vi "Collision Detection.vi"(2 "Map Entity Objects Positions":T3(array[cluster]), 3 "Max Player ID number":i32, 4 "Moving Object":T2) -> (0 "Bullet hit Player No.":i32, 1 "New Vector":T1)   [LabVIEW 2021]
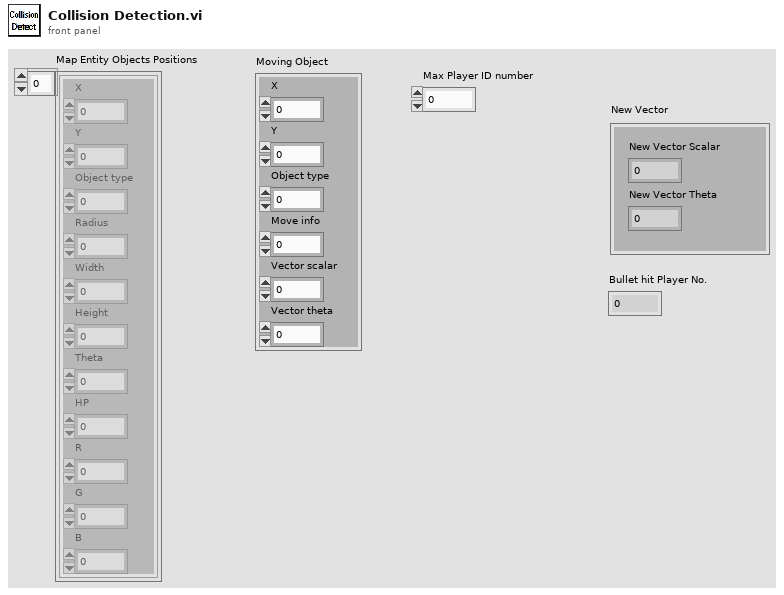
[diagram p1: front panel]
types:
  T1 = cluster{"New Vector Scalar":dbl, "New Vector Theta":dbl}
  T2 = cluster{"X":dbl, "Y":dbl, "Object type":dbl, "Move info":dbl, "Vector scalar":dbl, "Vector theta":dbl}
  T3 = cluster{"X":dbl, "Y":dbl, "Object type":dbl, "Radius":dbl, "Width":dbl, "Height":dbl, "Theta":dbl, "HP":dbl, "R":dbl, "G":dbl, "B":dbl}[]
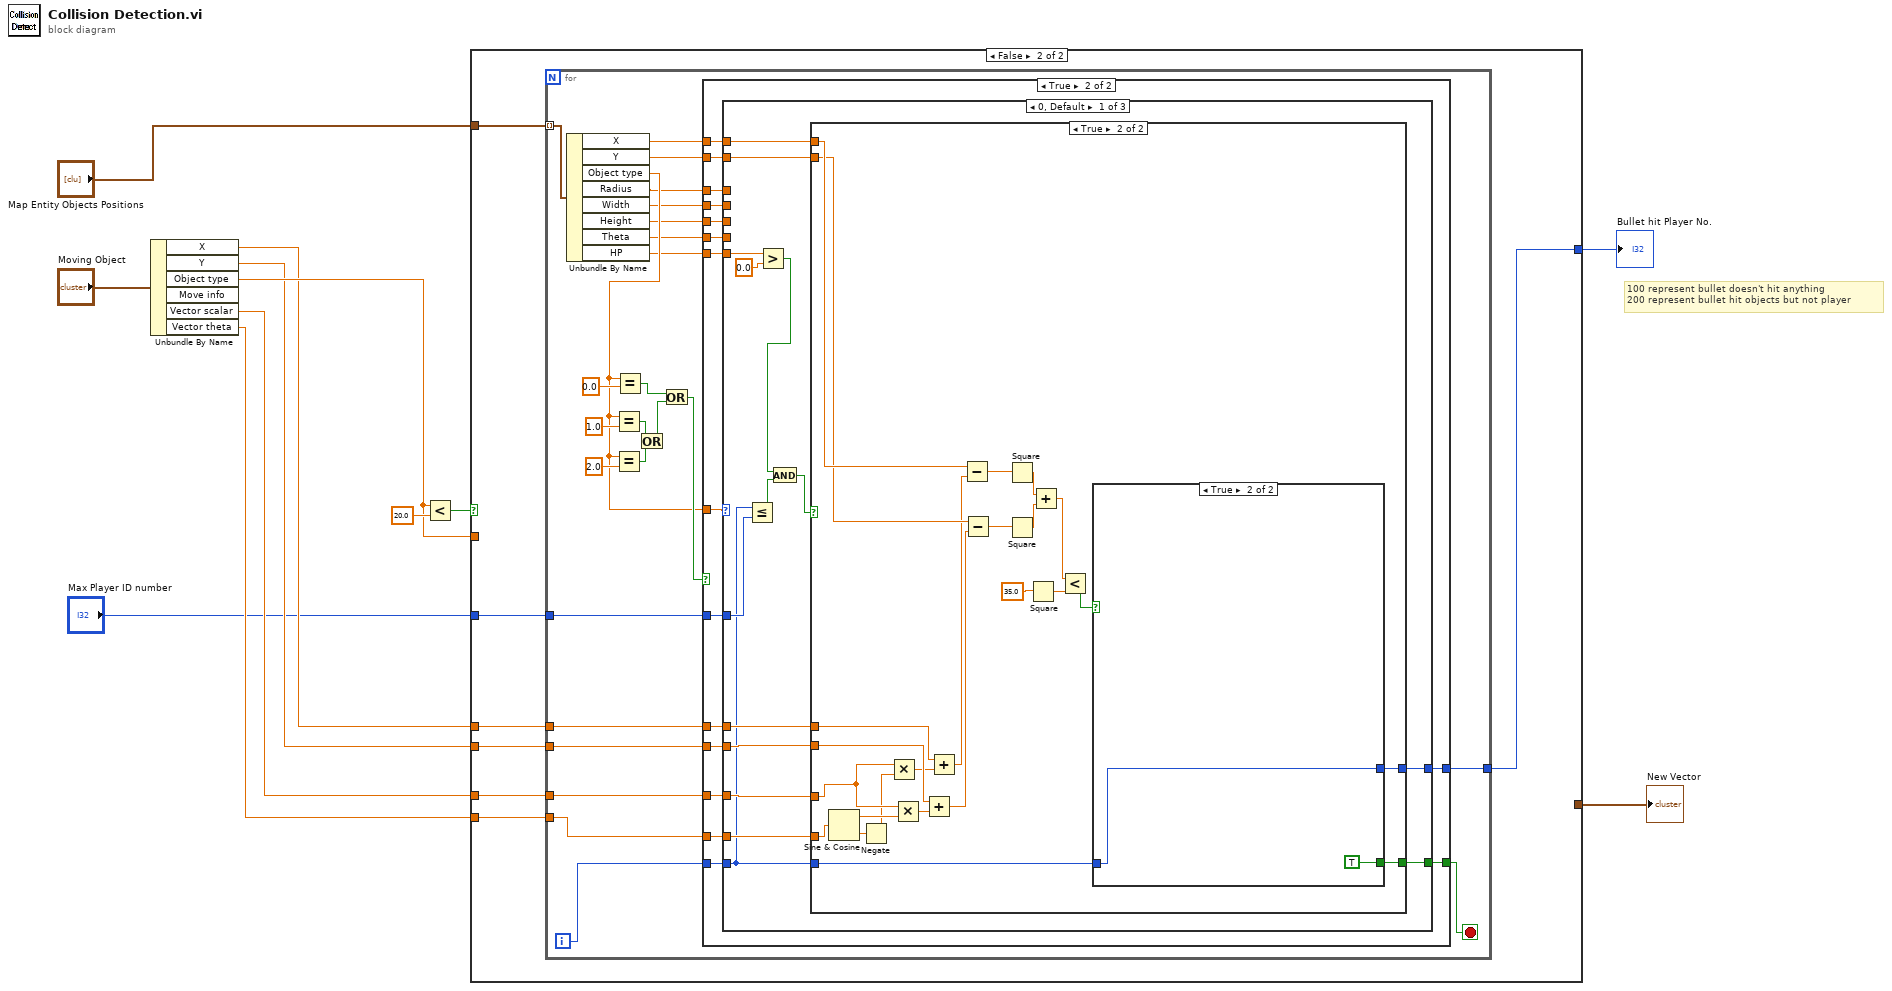
[diagram p0: block diagram]
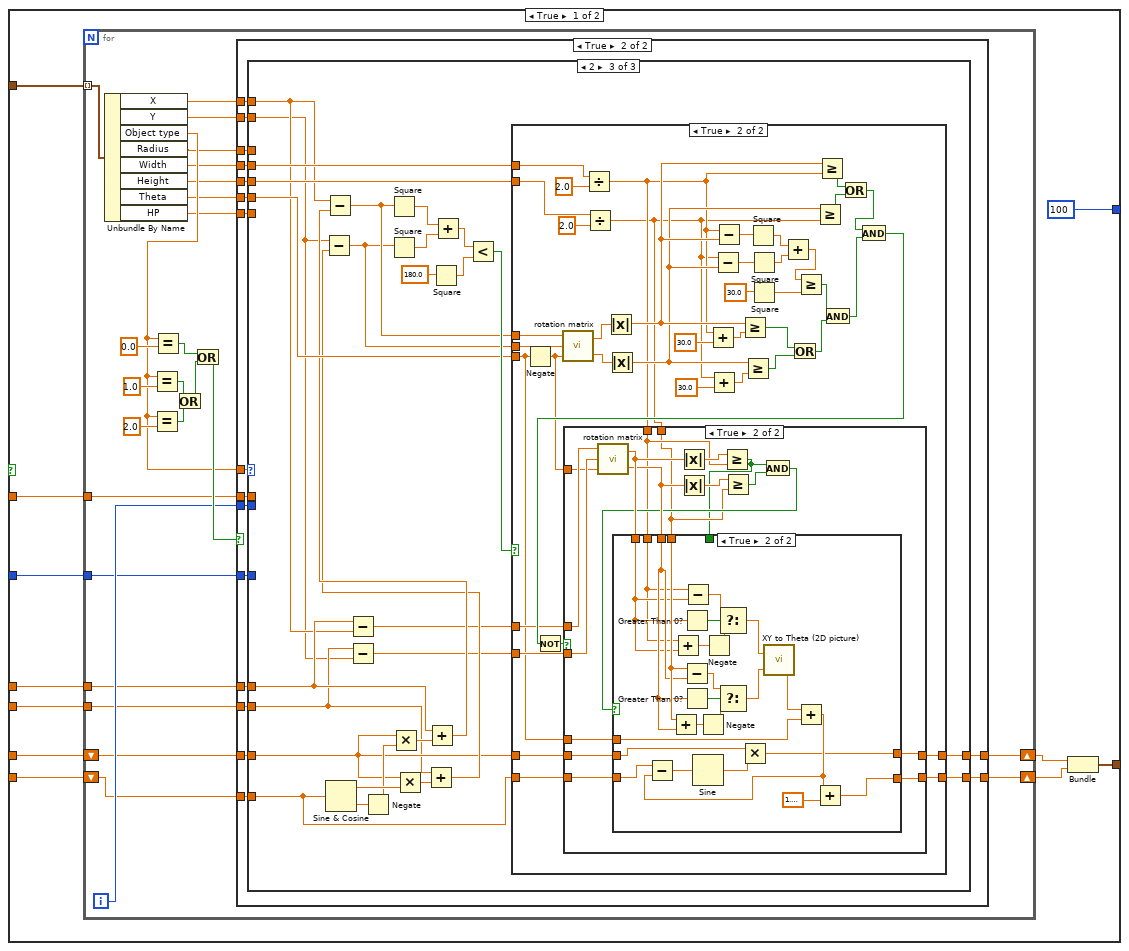
[diagram p2: hidden frame]
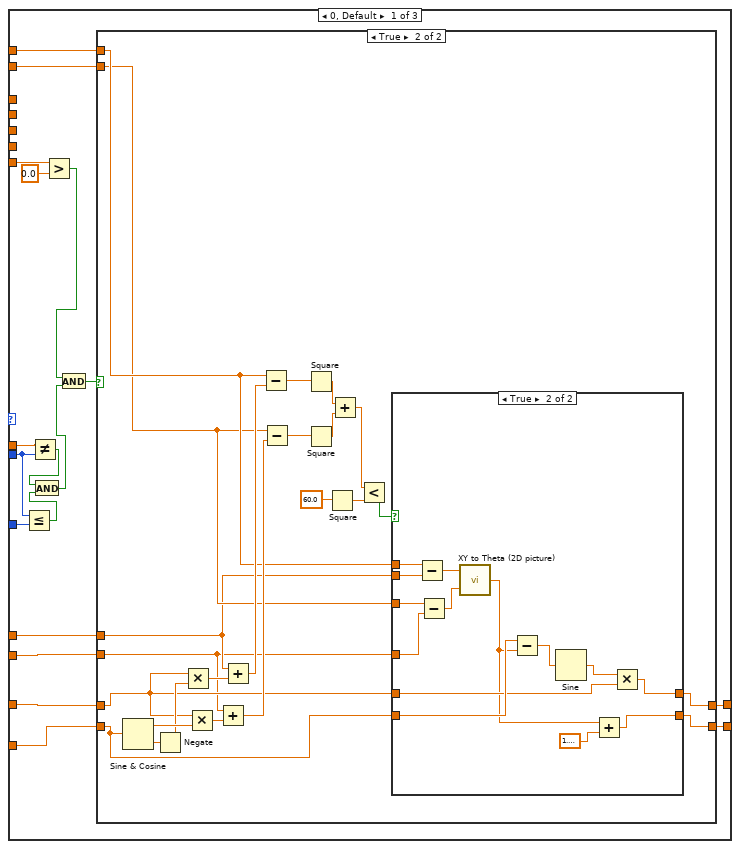
[diagram p4: hidden frame]
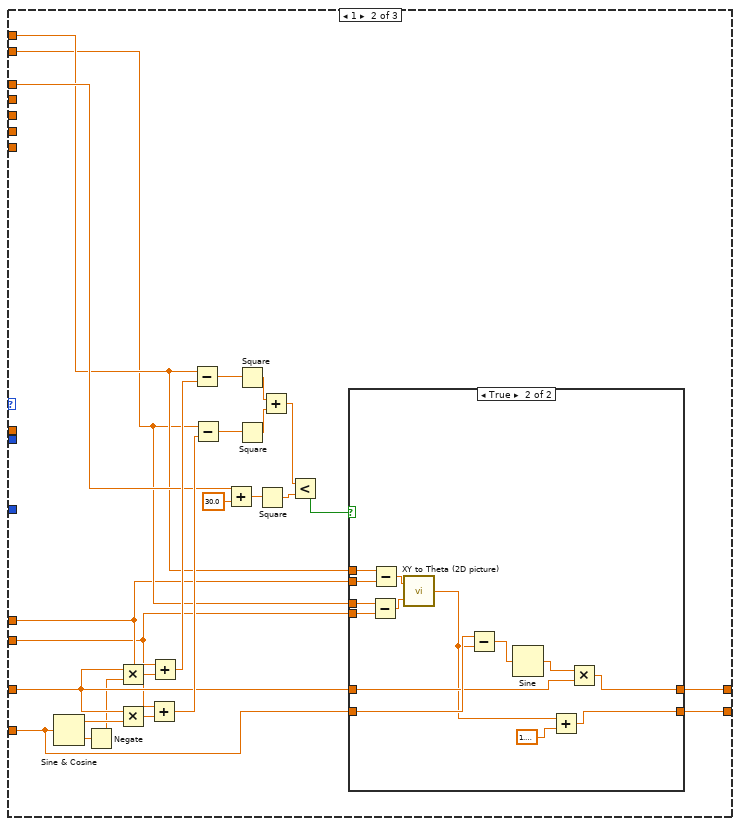
[diagram p7: hidden frame]
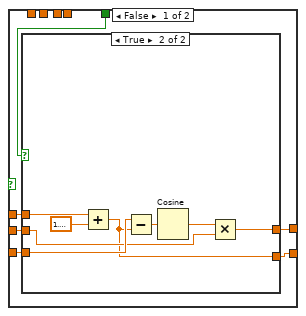
[diagram p11: hidden frame]
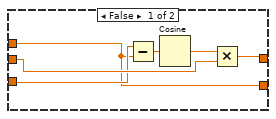
[diagram p12: hidden frame]
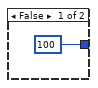
[diagram p13: hidden frame]
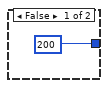
[diagram p14: hidden frame]
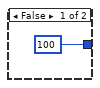
[diagram p15: hidden frame]
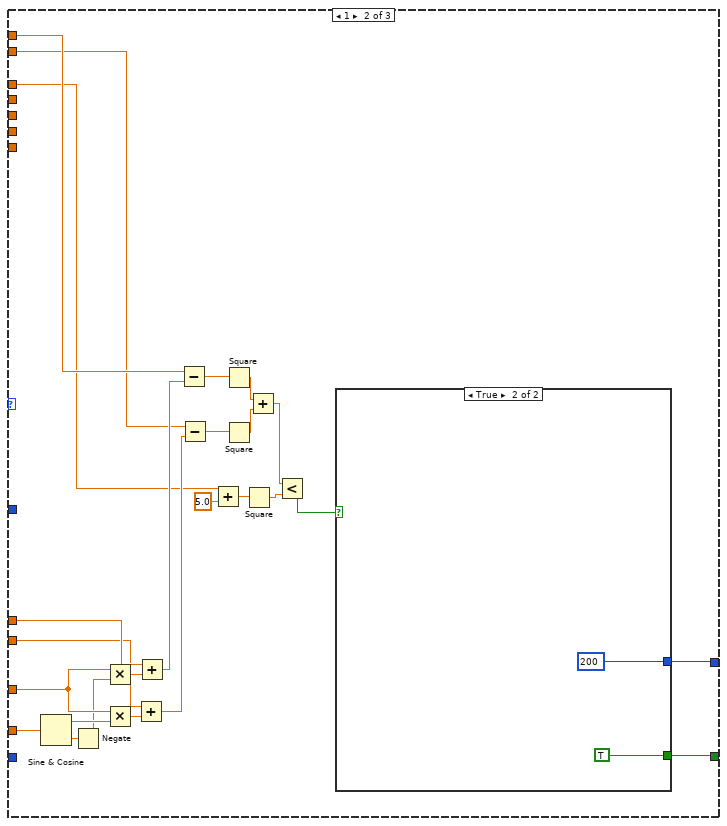
[diagram p16: hidden frame]
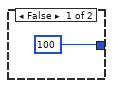
[diagram p17: hidden frame]
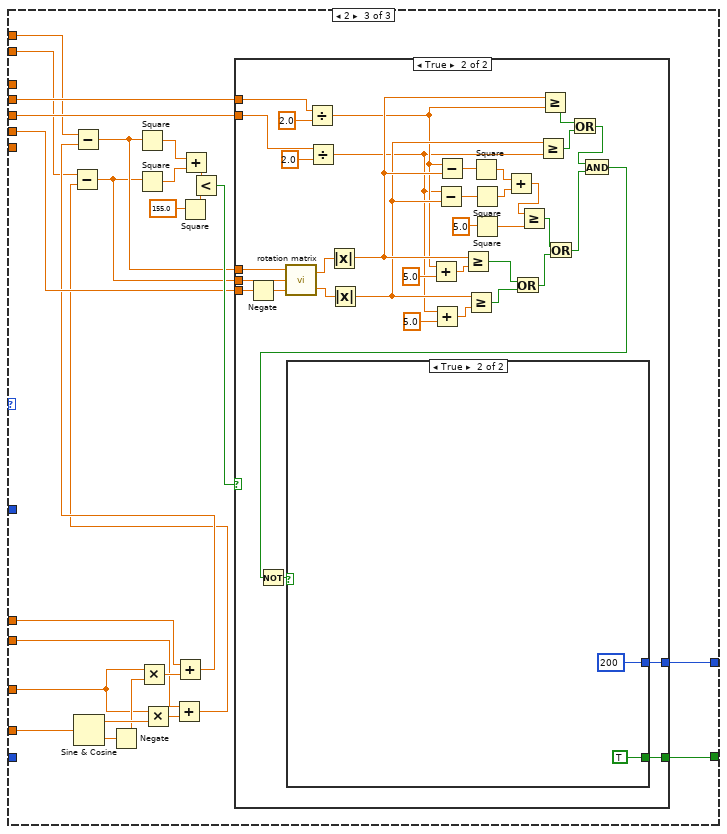
[diagram p18: hidden frame]
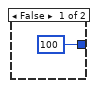
[diagram p19: hidden frame]
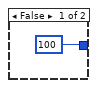
[diagram p20: hidden frame]
diagram:
  # "100 represent bullet doesn't hit anything\n200 represent bullet hit objects but not player"
  n1 = Unbundle By Name("Moving Object") -> ("X"=w4:dbl, "Y"=w3:dbl, "Object type"=w7:dbl, "Vector scalar"=w6:dbl, "Vector theta"=w5:dbl)  [unwired: 1 out]
  n2 = Less?(x=w7, y=20.0) -> (x < y?=w10:bool)
  n3 = case shown="False" w10 {
    tunnel: "Map Entity Objects Positions" -> [w23 w309]
    tunnel: [100 ("Bullet hit Player No.") w304] -> w8
    tunnel: w7 -> [w21 _]
    tunnel: w6 -> [w20 w308]
    tunnel: w5 -> [w19 w307]
    tunnel: w4 -> [w18 w306]
    tunnel: w3 -> [w17 w305]
    tunnel: [w14 _] -> w2
    tunnel: "Max Player ID number" -> [w13 w303]
    frame True {
      n4 = for {
        tunnel: w23 -> [w49] mode=indexing
        tunnel: w21 -> [w38]
        tunnel: w18 -> [w35]
        tunnel: w17 -> [w34]
        shift-right: [w30] -> w16
        shift-left: w20 -> [w36]
        shift-right: [w29] -> w15
        shift-left: w19 -> [w37]
        tunnel: w13 -> [w25]
        i -> [w39]
        n5 = Unbundle By Name(w49) -> ("X"=w33:dbl, "Y"=w32:dbl, "Object type"=w40:dbl, "Radius"=w31:dbl, "Width"=w28:dbl, "Height"=w27:dbl, "Theta"=w26:dbl, "HP"=w24:dbl)
        n6 = Equal?(x=w40, y=1.0) -> (x = y?=w45:bool)
        n7 = Equal?(x=w40, y=2.0) -> (x = y?=w44:bool)
        n8 = Equal?(x=w40, y=0.0) -> (x = y?=w43:bool)
        n9 = Or(x=w45, y=w44) -> (x .or. y?=w42:bool)
        n10 = Or(x=w43, y=w42) -> (x .or. y?=w41:bool)
        n11 = case shown="True" w41 {
          tunnel: w40 -> [_ w68]
          tunnel: w39 -> [_ w67]
          tunnel: w38 -> [_ w66]
          tunnel: w37 -> [w50 w65]
          tunnel: w36 -> [w51 w64]
          tunnel: w35 -> [_ w63]
          tunnel: w34 -> [_ w62]
          tunnel: w33 -> [_ w61]
          tunnel: w32 -> [_ w60]
          tunnel: w31 -> [_ w59]
          tunnel: [w51 w58] -> w30
          tunnel: [w50 w57] -> w29
          tunnel: w28 -> [_ w56]
          tunnel: w27 -> [_ w55]
          tunnel: w26 -> [_ w54]
          tunnel: w25 -> [_ w53]
          tunnel: w24 -> [_ w52]
          frame False {
          }
          frame True {
            n12 = case shown="2" w68 {
              tunnel: w67 -> [w75 _ _]
              tunnel: w66 -> [w86 _ _]
              tunnel: w65 -> [w82 w138 w176]
              tunnel: w64 -> [w84 w140 w175]
              tunnel: w63 -> [w80 w129 w172]
              tunnel: w62 -> [w81 w128 w170]
              tunnel: w61 -> [w79 w131 w171]
              tunnel: w60 -> [w78 w130 w169]
              tunnel: w59 -> [_ w143 _]
              tunnel: [w85 w141 w190] -> w58
              tunnel: [w83 w139 w189] -> w57
              tunnel: w56 -> [_ _ w178]
              tunnel: w55 -> [_ _ w177]
              tunnel: w54 -> [_ _ w186]
              tunnel: w53 -> [w74 _ _]
              tunnel: w52 -> [w73 _ _]
              frame 0, Default {
                n13 = Less Or Equal?(x=w75, y=w74) -> (x <= y?=w76:bool)
                n14 = Not Equal?(x=w86, y=w75) -> (x != y?=w77:bool)
                n15 = And(x=w77, y=w76) -> (x .and. y?=w69:bool)
                n16 = Greater?(x=w73, y=0.0) -> (0:w70:bool)
                n17 = And(x=w70, y=w69) -> (x .and. y?=w71:bool)
                n18 = case shown="True" w71 {
                  tunnel: [w88 w96] -> w85
                  tunnel: w84 -> [w88 w97]
                  tunnel: [w87 w95] -> w83
                  tunnel: w82 -> [w87 w98]
                  tunnel: w81 -> [_ w89]
                  tunnel: w80 -> [_ w90]
                  tunnel: w79 -> [_ w92]
                  tunnel: w78 -> [_ w91]
                  frame False {
                  }
                  frame True {
                    n19 = Sine & Cosine(0:w98) -> (1:w111:dbl, 2:w100:dbl)
                    n20 = Negate(x=w100) -> (-x=w99:dbl)
                    n21 = Multiply(x=w97, y=w99) -> (x*y=w109:dbl)
                    n22 = Multiply(x=w97, y=w111) -> (x*y=w110:dbl)
                    n23 = Add(x=w89, y=w110) -> (x+y=w108:dbl)
                    n24 = Add(x=w90, y=w109) -> (x+y=w107:dbl)
                    n25 = Subtract(x=w92, y=w107) -> (x-y=w102:dbl)
                    n26 = Subtract(x=w91, y=w108) -> (x-y=w101:dbl)
                    n27 = Square(x=w102) -> (x^2=w105:dbl)
                    n28 = Square(x=w101) -> (x^2=w106:dbl)
                    n29 = Square(x=60.0 ("y")) -> (x^2=w94:dbl)
                    n30 = Add(x=w105, y=w106) -> (x+y=w104:dbl)
                    n31 = Less?(x=w104, y=w94) -> (x < y?=w103:bool)
                    n32 = case shown="True" w103 {
                      tunnel: [w113 w126] -> w96
                      tunnel: w97 -> [w113 w123]
                      tunnel: [w112 w120] -> w95
                      tunnel: w98 -> [w112 w127]
                      tunnel: w92 -> [_ w117]
                      tunnel: w91 -> [_ w116]
                      tunnel: w90 -> [_ w115]
                      tunnel: w89 -> [_ w114]
                      frame False {
                      }
                      frame True {
                        n33 = Subtract(x=w117, y=w115) -> (x-y=w119:dbl)
                        n34 = Subtract(x=w116, y=w114) -> (x-y=w118:dbl)
                        n35 = call "XY to Theta (2D picture).vi"("y"=w118, "x"=w119) -> ("Theta"=w121:dbl)
                        n36 = Subtract(x=w127, y=w121) -> (x-y=w124:dbl)
                        n37 = Sine(x=w124) -> (sin(x)=w125:dbl)
                        n38 = Add(x=w121, y=1.5707963267948966) -> (x+y=w120:dbl)
                        n39 = Multiply(x=w125, y=w123) -> (x*y=w126:dbl)
                      }
                    }
                  }
                }
              }
              frame 1 {
                n40 = Sine & Cosine(0:w138) -> (1:w152:dbl, 2:w135:dbl)
                n41 = Negate(x=w135) -> (-x=w134:dbl)
                n42 = Multiply(x=w140, y=w134) -> (x*y=w150:dbl)
                n43 = Multiply(x=w140, y=w152) -> (x*y=w151:dbl)
                n44 = Add(x=w128, y=w151) -> (x+y=w149:dbl)
                n45 = Add(x=w129, y=w150) -> (x+y=w148:dbl)
                n46 = Subtract(x=w131, y=w148) -> (x-y=w137:dbl)
                n47 = Subtract(x=w130, y=w149) -> (x-y=w136:dbl)
                n48 = Add(x=w143, y=30.0) -> (x+y=w132:dbl)
                n49 = Square(x=w137) -> (x^2=w146:dbl)
                n50 = Square(x=w136) -> (x^2=w147:dbl)
                n51 = Square(x=w132) -> (x^2=w133:dbl)
                n52 = Add(x=w146, y=w147) -> (x+y=w145:dbl)
                n53 = Less?(x=w145, y=w133) -> (x < y?=w142:bool)
                n54 = case shown="True" w142 {
                  tunnel: [w154 w167] -> w141
                  tunnel: w140 -> [w154 w164]
                  tunnel: [w153 w161] -> w139
                  tunnel: w138 -> [w153 w168]
                  tunnel: w131 -> [_ w158]
                  tunnel: w130 -> [_ w157]
                  tunnel: w129 -> [_ w156]
                  tunnel: w128 -> [_ w155]
                  frame False {
                  }
                  frame True {
                    n55 = Subtract(x=w157, y=w155) -> (x-y=w160:dbl)
                    n56 = Subtract(x=w158, y=w156) -> (x-y=w159:dbl)
                    n57 = call "XY to Theta (2D picture).vi"("y"=w160, "x"=w159) -> ("Theta"=w162:dbl)
                    n58 = Subtract(x=w168, y=w162) -> (x-y=w165:dbl)
                    n59 = Sine(x=w165) -> (sin(x)=w166:dbl)
                    n60 = Add(x=w162, y=1.5707963267948966) -> (x+y=w161:dbl)
                    n61 = Multiply(x=w166, y=w164) -> (x*y=w167:dbl)
                  }
                }
              }
              frame 2 {
                n62 = Sine & Cosine(0:w176) -> (1:w185:dbl, 2:w182:dbl)
                n63 = Subtract(x=w172, y=w171) -> (x-y=w174:dbl)
                n64 = Subtract(x=w170, y=w169) -> (x-y=w173:dbl)
                n65 = Negate(x=w182) -> (-x=w181:dbl)
                n66 = Multiply(x=w175, y=w181) -> (x*y=w183:dbl)
                n67 = Multiply(x=w175, y=w185) -> (x*y=w184:dbl)
                n68 = Add(x=w170, y=w184) -> (x+y=w179:dbl)
                n69 = Subtract(x=w169, y=w179) -> (x-y=w187:dbl)
                n70 = Square(x=w187) -> (x^2=w196:dbl)
                n71 = Add(x=w172, y=w183) -> (x+y=w180:dbl)
                n72 = Subtract(x=w171, y=w180) -> (x-y=w188:dbl)
                n73 = Square(x=w188) -> (x^2=w195:dbl)
                n74 = Square(x=180.0 ("y")) -> (x^2=w192:dbl)
                n75 = Add(x=w195, y=w196) -> (x+y=w194:dbl)
                n76 = Less?(x=w194, y=w192) -> (x < y?=w191:bool)
                n77 = case shown="True" w191 {
                  tunnel: [w198 w212] -> w190
                  tunnel: w175 -> [w198 w211]
                  tunnel: [w197 w210] -> w189
                  tunnel: w176 -> [w197 w209]
                  tunnel: w188 -> [_ w239]
                  tunnel: w187 -> [_ w238]
                  tunnel: w186 -> [_ w203]
                  tunnel: w178 -> [_ w235]
                  tunnel: w177 -> [_ w234]
                  tunnel: w174 -> [_ w208]
                  tunnel: w173 -> [_ w207]
                  frame False {
                  }
                  frame True {
                    n78 = Negate(x=w203) -> (-x=w206:dbl)
                    n79 = call "rotation matrix.vi"("angle"=w206, "y"=w238, "x"=w239) -> ("new y"=w232:dbl, "new x"=w233:dbl)
                    n80 = Divide(x=w235, y=2.0) -> (x/y=w205:dbl)
                    n81 = Divide(x=w234, y=2.0) -> (x/y=w204:dbl)
                    n82 = Absolute Value(x=w233) -> (abs(x)=w216:dbl)
                    n83 = Absolute Value(x=w232) -> (abs(x)=w215:dbl)
                    n84 = Add(x=w205, y=30.0) -> (x+y=w226:dbl)
                    n85 = Add(x=w204, y=30.0) -> (x+y=w227:dbl)
                    n86 = Subtract(x=w204, y=w215) -> (x-y=w217:dbl)
                    n87 = Subtract(x=w205, y=w216) -> (x-y=w218:dbl)
                    n88 = Greater Or Equal?(x=w216, y=w226) -> (x >= y?=w231:bool)
                    n89 = Greater Or Equal?(x=w215, y=w227) -> (x >= y?=w230:bool)
                    n90 = Square(x=w218) -> (x^2=w221:dbl)
                    n91 = Square(x=w217) -> (x^2=w220:dbl)
                    n92 = Square(x=30.0 ("y")) -> (x^2=w225:dbl)
                    n93 = Add(x=w221, y=w220) -> (x+y=w219:dbl)
                    n94 = Or(x=w231, y=w230) -> (x .or. y?=w199:bool)
                    n95 = Greater Or Equal?(x=w219, y=w225) -> (x >= y?=w223:bool)
                    n96 = Greater Or Equal?(x=w215, y=w204) -> (x >= y?=w202:bool)
                    n97 = Greater Or Equal?(x=w216, y=w205) -> (x >= y?=w201:bool)
                    n98 = And(x=w223, y=w199) -> (x .and. y?=w222:bool)
                    n99 = Or(x=w201, y=w202) -> (x .or. y?=w200:bool)
                    n100 = And(x=w200, y=w222) -> (x .and. y?=w213:bool)
                    n101 = Not(x=w213) -> (.not. x?=w214:bool)
                    n102 = case shown="True" w214 {
                      tunnel: [w241 w245] -> w212
                      tunnel: w211 -> [w241 w243]
                      tunnel: [w240 w246] -> w210
                      tunnel: w209 -> [w240 w244]
                      tunnel: w208 -> [_ w258]
                      tunnel: w207 -> [_ w257]
                      tunnel: w206 -> [_ w256]
                      tunnel: w205 -> [_ w249]
                      tunnel: w204 -> [_ w248]
                      tunnel: w203 -> [_ w247]
                      frame False {
                      }
                      frame True {
                        n103 = call "rotation matrix.vi"("angle"=w256, "y"=w257, "x"=w258) -> ("new y"=w254:dbl, "new x"=w255:dbl)
                        n104 = Absolute Value(x=w255) -> (abs(x)=w250:dbl)
                        n105 = Absolute Value(x=w254) -> (abs(x)=w251:dbl)
                        n106 = Greater Or Equal?(x=w250, y=w249) -> (x >= y?=w242:bool)
                        n107 = Greater Or Equal?(x=w251, y=w248) -> (x >= y?=w253:bool)
                        n108 = And(x=w242, y=w253) -> (x .and. y?=w252:bool)
                        n109 = case shown="True" w252 {
                          tunnel: w254 -> [_ w297]
                          tunnel: w248 -> [_ w298]
                          tunnel: w255 -> [_ w296]
                          tunnel: w249 -> [_ w282]
                          tunnel: w247 -> [w263 w292]
                          tunnel: [w259 w290] -> w246
                          tunnel: [w260 w284] -> w245
                          tunnel: w244 -> [w262 w289]
                          tunnel: w243 -> [w261 w285]
                          tunnel: w242 -> [w264 _]
                          frame False {
                            n110 = case shown="True" w264 {
                              tunnel: w263 -> [w265 w277]
                              tunnel: w262 -> [w266 w276]
                              tunnel: w261 -> [w267 w274]
                              tunnel: [w268 w272] -> w260
                              tunnel: [w265 w271] -> w259
                              frame False {
                                n111 = Subtract(x=w266, y=w265) -> (x-y=w270:dbl)
                                n112 = Cosine(x=w270) -> (cos(x)=w269:dbl)
                                n113 = Multiply(x=w269, y=w267) -> (x*y=w268:dbl)
                              }
                              frame True {
                                n114 = Add(x=w277, y=1.5707963267948966) -> (x+y=w271:dbl)
                                n115 = Subtract(x=w276, y=w271) -> (x-y=w275:dbl)
                                n116 = Cosine(x=w275) -> (cos(x)=w273:dbl)
                                n117 = Multiply(x=w273, y=w274) -> (x*y=w272:dbl)
                              }
                            }
                          }
                          frame True {
                            n118 = Add(x=w298, y=w297) -> (x+y=w280:dbl)
                            n119 = Add(x=w282, y=w296) -> (x+y=w279:dbl)
                            n120 = Greater Than 0?(x=w296) -> (x > 0?=w299:bool)
                            n121 = Subtract(x=w298, y=w297) -> (x-y=w302:dbl)
                            n122 = Greater Than 0?(x=w297) -> (x > 0?=w300:bool)
                            n123 = Subtract(x=w282, y=w296) -> (x-y=w301:dbl)
                            n124 = Negate(x=w280) -> (-x=w281:dbl)
                            n125 = Negate(x=w279) -> (-x=w283:dbl)
                            n126 = Select(t=w301, s=w299, f=w283) -> (s? t:f=w295:dbl)
                            n127 = Select(t=w302, s=w300, f=w281) -> (s? t:f=w294:dbl)
                            n128 = call "XY to Theta (2D picture).vi"("y"=w294, "x"=w295) -> ("Theta"=w293:dbl)
                            n129 = Add(x=w293, y=w292) -> (x+y=w288:dbl)
                            n130 = Subtract(x=w289, y=w288) -> (x-y=w287:dbl)
                            n131 = Sine(x=w287) -> (sin(x)=w286:dbl)
                            n132 = Multiply(x=w285, y=w286) -> (x*y=w284:dbl)
                            n133 = Add(x=w288, y=1.5707963267948966) -> (x+y=w290:dbl)
                          }
                        }
                      }
                    }
                  }
                }
              }
            }
          }
        }
      }
      n134 = Bundle("Vector scalar"=w16, "Vector theta"=w15) -> (w14:cluster{"Vector scalar":dbl, "Vector theta":dbl})  [unwired: 1 in]
    }
    frame False {
      n135 = for {
        tunnel: w309 -> [w334] mode=indexing
        tunnel: w306 -> [w322]
        tunnel: w305 -> [w321]
        tunnel: w308 -> [w323]
        tunnel: w307 -> [w324]
        tunnel: [w312] -> w304
        tunnel: w303 -> [w311]
        i -> [w313]
        stop <- w314 stop-if-true
        n136 = Unbundle By Name(w334) -> ("X"=w320:dbl, "Y"=w319:dbl, "Object type"=w325:dbl, "Radius"=w318:dbl, "Width"=w317:dbl, "Height"=w316:dbl, "Theta"=w315:dbl, "HP"=w310:dbl)
        n137 = Equal?(x=w325, y=1.0) -> (x = y?=w330:bool)
        n138 = Equal?(x=w325, y=2.0) -> (x = y?=w329:bool)
        n139 = Equal?(x=w325, y=0.0) -> (x = y?=w328:bool)
        n140 = Or(x=w330, y=w329) -> (x .or. y?=w327:bool)
        n141 = Or(x=w328, y=w327) -> (x .or. y?=w326:bool)
        n142 = case shown="True" w326 {
          tunnel: w325 -> [_ w351]
          tunnel: w324 -> [_ w350]
          tunnel: w323 -> [_ w349]
          tunnel: w322 -> [_ w348]
          tunnel: w321 -> [_ w347]
          tunnel: w320 -> [_ w346]
          tunnel: w319 -> [_ w345]
          tunnel: w318 -> [_ w344]
          tunnel: w317 -> [_ w343]
          tunnel: w316 -> [_ w342]
          tunnel: w315 -> [_ w341]
          tunnel: [_ w340] -> w314
          tunnel: w313 -> [_ w339]
          tunnel: [100 w338] -> w312
          tunnel: w311 -> [_ w337]
          tunnel: w310 -> [_ w336]
          frame False {
          }
          frame True {
            n143 = case shown="0, Default" w351 {
              tunnel: w350 -> [w365 w403 w430]
              tunnel: w349 -> [w366 w404 w429]
              tunnel: w348 -> [w363 w416 w428]
              tunnel: w347 -> [w364 w415 w426]
              tunnel: w346 -> [w362 w412 w427]
              tunnel: w345 -> [w361 w411 w425]
              tunnel: w344 -> [_ w406 _]
              tunnel: w343 -> [_ _ w432]
              tunnel: w342 -> [_ _ w431]
              tunnel: w341 -> [_ _ w440]
              tunnel: [w360 w395 w424] -> w340
              tunnel: w339 -> [w357 _ _]
              tunnel: [w359 w396 w423] -> w338
              tunnel: w337 -> [w358 _ _]
              tunnel: w336 -> [w355 _ _]
              frame 0, Default {
                n144 = Less Or Equal?(x=w357, y=w358) -> (x <= y?=w353:bool)
                n145 = Greater?(x=w355, y=0.0) -> (0:w354:bool)
                n146 = And(x=w354, y=w353) -> (x .and. y?=w352:bool)
                n147 = case shown="True" w352 {
                  tunnel: w366 -> [_ w391]
                  tunnel: w365 -> [_ w390]
                  tunnel: w364 -> [_ w389]
                  tunnel: w363 -> [_ w388]
                  tunnel: w362 -> [_ w387]
                  tunnel: w361 -> [_ w386]
                  tunnel: [_ w370] -> w360
                  tunnel: w357 -> [_ w369]
                  tunnel: [200 w368] -> w359
                  frame False {
                  }
                  frame True {
                    n148 = Sine & Cosine(0:w390) -> (1:w385:dbl, 2:w374:dbl)
                    n149 = Negate(x=w374) -> (-x=w373:dbl)
                    n150 = Multiply(x=w391, y=w373) -> (x*y=w383:dbl)
                    n151 = Multiply(x=w391, y=w385) -> (x*y=w384:dbl)
                    n152 = Add(x=w389, y=w384) -> (x+y=w382:dbl)
                    n153 = Add(x=w388, y=w383) -> (x+y=w381:dbl)
                    n154 = Subtract(x=w387, y=w381) -> (x-y=w376:dbl)
                    n155 = Subtract(x=w386, y=w382) -> (x-y=w375:dbl)
                    n156 = Square(x=w376) -> (x^2=w379:dbl)
                    n157 = Square(x=w375) -> (x^2=w380:dbl)
                    n158 = Square(x=35.0 ("y")) -> (x^2=w372:dbl)
                    n159 = Add(x=w379, y=w380) -> (x+y=w378:dbl)
                    n160 = Less?(x=w378, y=w372) -> (x < y?=w377:bool)
                    n161 = case shown="True" w377 {
                      tunnel: [_ TRUE] -> w370
                      tunnel: w369 -> [_ w393]
                      tunnel: [100 w393] -> w368
                      frame False {
                      }
                      frame True {
                      }
                    }
                  }
                }
              }
              frame 1 {
                n162 = Sine & Cosine(0:w403) -> (1:w419:dbl, 2:w400:dbl)
                n163 = Negate(x=w400) -> (-x=w399:dbl)
                n164 = Multiply(x=w404, y=w399) -> (x*y=w417:dbl)
                n165 = Multiply(x=w404, y=w419) -> (x*y=w418:dbl)
                n166 = Add(x=w415, y=w418) -> (x+y=w414:dbl)
                n167 = Add(x=w416, y=w417) -> (x+y=w413:dbl)
                n168 = Subtract(x=w412, y=w413) -> (x-y=w402:dbl)
                n169 = Subtract(x=w411, y=w414) -> (x-y=w401:dbl)
                n170 = Add(x=w406, y=5.0) -> (x+y=w397:dbl)
                n171 = Square(x=w402) -> (x^2=w409:dbl)
                n172 = Square(x=w401) -> (x^2=w410:dbl)
                n173 = Square(x=w397) -> (x^2=w398:dbl)
                n174 = Add(x=w409, y=w410) -> (x+y=w408:dbl)
                n175 = Less?(x=w408, y=w398) -> (x < y?=w405:bool)
                n176 = case shown="True" w405 {
                  tunnel: [100 200] -> w396
                  tunnel: [_ TRUE] -> w395
                  frame False {
                  }
                  frame True {
                  }
                }
              }
              frame 2 {
                n177 = Sine & Cosine(0:w430) -> (1:w439:dbl, 2:w436:dbl)
                n178 = Negate(x=w436) -> (-x=w435:dbl)
                n179 = Multiply(x=w429, y=w435) -> (x*y=w437:dbl)
                n180 = Multiply(x=w429, y=w439) -> (x*y=w438:dbl)
                n181 = Add(x=w426, y=w438) -> (x+y=w433:dbl)
                n182 = Subtract(x=w425, y=w433) -> (x-y=w441:dbl)
                n183 = Square(x=w441) -> (x^2=w448:dbl)
                n184 = Add(x=w428, y=w437) -> (x+y=w434:dbl)
                n185 = Subtract(x=w427, y=w434) -> (x-y=w442:dbl)
                n186 = Square(x=w442) -> (x^2=w447:dbl)
                n187 = Square(x=155.0 ("y")) -> (x^2=w444:dbl)
                n188 = Add(x=w447, y=w448) -> (x+y=w446:dbl)
                n189 = Less?(x=w446, y=w444) -> (x < y?=w443:bool)
                n190 = case shown="True" w443 {
                  tunnel: w442 -> [_ w486]
                  tunnel: w441 -> [_ w485]
                  tunnel: w440 -> [_ w452]
                  tunnel: w432 -> [_ w482]
                  tunnel: w431 -> [_ w481]
                  tunnel: [_ w451] -> w424
                  tunnel: [100 w450] -> w423
                  frame False {
                  }
                  frame True {
                    n191 = Negate(x=w452) -> (-x=w455:dbl)
                    n192 = call "rotation matrix.vi"("angle"=w455, "y"=w485, "x"=w486) -> ("new y"=w479:dbl, "new x"=w480:dbl)
                    n193 = Divide(x=w482, y=2.0) -> (x/y=w454:dbl)
                    n194 = Divide(x=w481, y=2.0) -> (x/y=w453:dbl)
                    n195 = Absolute Value(x=w480) -> (abs(x)=w459:dbl)
                    n196 = Absolute Value(x=w479) -> (abs(x)=w458:dbl)
                    n197 = Add(x=w454, y=5.0) -> (x+y=w473:dbl)
                    n198 = Add(x=w453, y=5.0) -> (x+y=w474:dbl)
                    n199 = Subtract(x=w453, y=w458) -> (x-y=w460:dbl)
                    n200 = Subtract(x=w454, y=w459) -> (x-y=w461:dbl)
                    n201 = Greater Or Equal?(x=w459, y=w473) -> (x >= y?=w478:bool)
                    n202 = Greater Or Equal?(x=w458, y=w474) -> (x >= y?=w477:bool)
                    n203 = Square(x=w461) -> (x^2=w464:dbl)
                    n204 = Square(x=w460) -> (x^2=w463:dbl)
                    n205 = Square(x=5.0 ("y")) -> (x^2=w472:dbl)
                    n206 = Add(x=w464, y=w463) -> (x+y=w462:dbl)
                    n207 = Or(x=w478, y=w477) -> (x .or. y?=w470:bool)
                    n208 = Greater Or Equal?(x=w462, y=w472) -> (x >= y?=w469:bool)
                    n209 = Greater Or Equal?(x=w458, y=w453) -> (x >= y?=w466:bool)
                    n210 = Greater Or Equal?(x=w459, y=w454) -> (x >= y?=w467:bool)
                    n211 = Or(x=w469, y=w470) -> (x .or. y?=w468:bool)
                    n212 = Or(x=w467, y=w466) -> (x .or. y?=w465:bool)
                    n213 = And(x=w465, y=w468) -> (x .and. y?=w456:bool)
                    n214 = Not(x=w456) -> (.not. x?=w457:bool)
                    n215 = case shown="True" w457 {
                      tunnel: [_ TRUE] -> w451
                      tunnel: [100 200] -> w450
                      frame False {
                      }
                      frame True {
                      }
                    }
                  }
                }
              }
            }
          }
        }
      }
    }
  }
  "New Vector" <- w2
  "Bullet hit Player No." <- w8
